vi "Basic Spectral Measurement.vi"() -> ()   [LabVIEW 2011]
doc: "This example shows how to take a spectral measurement on a simulated signal. The spectral measurement is an Peak FFT of the simulated signal.\n\nThis example uses the following Express VIs: Simulate Signal and Spectral Measurements."
uses:
  Instance           1 34Saved   Basic Spectral Measurement .vi
  Instance           2 34Saved   Basic Spectral Measurement .vi
  <vilib>/express/express analysis/Spectral/Block/exnSpectralBlock spectral measurements peak poly.vi
  <vilib>/express/express analysis/Spectral/Block/exnSpectralBlock spectral measurements peak DDT.vi
  <vilib>/express/express analysis/Spectral/XNode/ExpressSpectralMeasurementsBlockNode.xnode
panel:
  in  "Frequency":dbl(slide)=100.49261083743842 scale=0.0..400.0
  out "Input":dynamicdata(graph)=[{"t0"=timestamp(21.300000190734863 s since 1904-01-01), "dt"=0.001, "Y"=[-1.045426032151304, -2.5037197611687847, -2.99654825251707, -2.3338707580624307, -0.7712238975993304, 1.0888164152541084, 2.5289956815818373, 2.9939630034054576, 2.304421243387486, 0.7262662136486071, -1.1319460307379796, -2.5536659166167683, -2.990660710912945, -2.2744198281053865, -0.6811345915494608, 1.1748045492149866, 2.5777245578409334, 2.9866421659267184, 2.2438736974472886, 0.6358398401632068, -1.2173817062239638, -2.6011658432962133, -2.981908330873862, -2.2127901671017156, -0.5903928074200355, 1.2596673046888083, 2.6239841588789767, 2.976460339490859, 2.1811766814624987, 0.5448043777209927, -1.3016512173606245, -2.6461740396846314, -2.9702994965520713, -2.149040811845846, -0.49908546933116904, 1.343323389243197, 2.6677301713164625, 2.9634272775572437, 2.116390254677054, 0.4532470317648392, -1.3846738400011034, -2.688647391158405, -2.9558453283781305, -2.0832328296472395, -0.4073000431630859, 1.4256926663499743, 2.708920689611468, 2.9475554648643163, 2.0495764778405503, 0.36125550766457465, -1.4663700444282954, -2.728545211293523, -2.9385596724083207, -2.015429259832296, -0.31512445277009044, 1.5066962321501958, 2.74751625620215, 2.928860105470117, 1.980799353758502, 0.2689179267015383, -1.5466615715386023, -2.7658292808402525, -2.91845908706113, -1.9456950533572277, -0.22264699575586266, 1.5862564910383523, 2.7834798993042416, 2.9073591081878947, 1.9101247659822758, 0.17632274165475645, -1.6254715078085045, -2.800463884334419, -2.895562827255464, -1.8740970105896557, -0.1299562588906167, 1.6642972299934566, 2.8167771683274005, 2.8830730694307336, 1.8376204156973226, 0.08355865206945358, -1.7027243589722605, -2.8324158443102894, -2.869892825965822, -1.8007037173186797, -0.03714103325137693, 1.7407436915856087, 2.8473761668763835, 2.8560252534816772, 1.763355756870333, -0.009285480710701972, -1.7783461223399577, -2.8616545530821855, -2.841473673212078, -1.725585479054605, 0.05570977083351682, 1.8155226455882614, 2.875247583305507, 2.8262415702082104, 1.68740192971731, -0.10212071866640285], "attributes"=variant("NI_ChannelName"=variant(string "Sine"), "NI_ExpIsRelativeTime"=variant(bool TRUE), "NI_ExpStartTimeStamp"=variant(dbl 3101836871.808), "NI_ExpTimeStamp"=variant(dbl 3101836893.1080003), "NI_ExpXDimension"=variant(string "t"))}]
  in  "stop":bool
  out "Result":dynamicdata(graph)=[{"t0"=timestamp(0 s since 1904-01-01), "dt"=10.0, "Y"=[0.00010119358321722769, 0.0001714924870246386, 0.00025292122341500343, 0.00039810034485058204, 0.000657349221237452, 0.00116806578140715, 0.0023425582433223473, 0.0058018715568664714, 0.022436898544568123, 1.3896389830932006, 2.995317296929077, 1.6111044258798126, 0.026903743652726436, 0.006478779647200742, 0.00255578447258286, 0.0012693725703337795, 0.0007229845347943666, 0.000451281491135843, 0.0003008497690725818, 0.0002107740678172362, 0.00015351123544835472, 0.00011534373387854474, 8.89073098943249e-05, 7.000352023481012e-05, 5.611775822605156e-05, 4.5680495495198856e-05, 3.767714283893824e-05, 3.1431752271894555e-05, 2.6482007367919793e-05, 2.2504325731545272e-05, 1.926755012813675e-05, 1.660350944705928e-05, 1.438783631069607e-05, 1.2527189117138286e-05, 1.0950570227509764e-05, 9.60332175204098e-06, 8.442907232564713e-06, 7.4359074645799366e-06, 6.555857664025357e-06, 5.781680061653417e-06, 5.096549315892468e-06, 4.487085322078512e-06, 3.942810128887706e-06, 3.4558405839675615e-06, 3.0208210345184687e-06, 2.6351310465532935e-06, 2.29941391720033e-06, 2.0183889589474995e-06, 1.8015353111065941e-06, 1.6623311196560747e-06], "attributes"=variant("NI_ChannelName"=variant(string "Sine"), "NI_ExpIsRelativeTime"=variant(bool TRUE), "NI_ExpStartTimeStamp"=variant(dbl 3101836871.808), "NI_ExpTimeStamp"=variant(dbl 3101836893.1080003), "NI_ExpXDimension"=variant(string "f"))}]
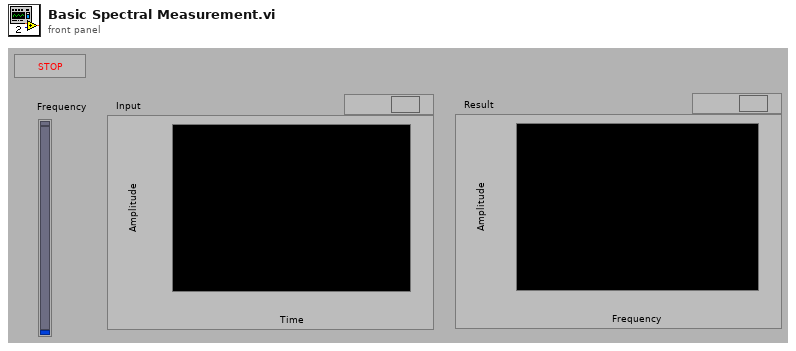
[diagram p1: front panel]
types:
  T1 = cluster{"averaging mode":u16, "weighting mode":u16, "number of averages":u32}
  T2 = cluster{"dB On (F)":bool, "unwrap phase (F)":bool, "convert to degree (F)":bool}
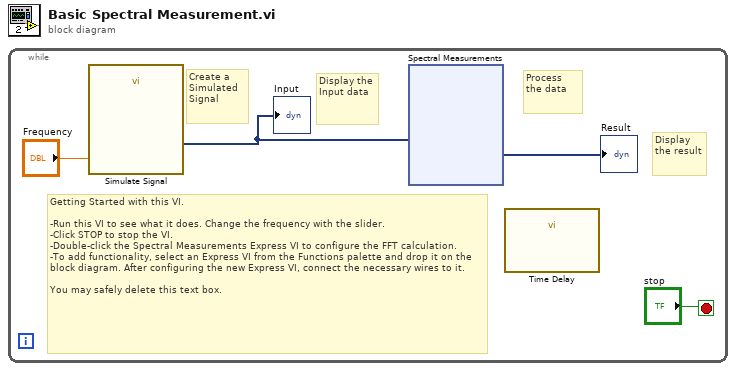
[diagram p0: block diagram]
diagram:
  n1 = while {
    stop <- "stop" stop-if-true
    # "Getting Started with this VI.\n\n-Run this VI to see what it does. Change the frequency with the slider.\n-Click STOP to stop the VI.\n-Double-click the Spectral Measurements Express VI to configure the FFT calculation.\n-To add functionality, select an Express VI from the Functions palette and drop it on the block diagram. After configuring the new Express VI, connect the necessary wires to it.\n\nYou may safely delete this text box."
    # "Display the Input data"
    # "Create a Simulated Signal"
    # "Process the data"
    # "Display the result"
    n2 = call "Simulate Signal"("Frequency"="Frequency") -> ("Sine"=w2:dynamicdata)  [unwired: 5 in, 9 out]
    "Input" <- w2
    n3 = xnode "Spectral Measurements"("Signals"=w2) -> ("FFT - (Peak)"=→"Result":dynamicdata)  [unwired: 1 in, 2 out]
    n4 = call "Time Delay"() -> ()  [unwired: 2 in, 10 out]
  }
